vi "OpenGDS_Installer.vi"() -> ()   [LabVIEW 2012]
uses:
  OpenGDS_Installer_State.ctl
  <vilib>/Utility/config.llb/Read Key (String).vi
  <vilib>/zip/NI_Unzip.lvlib
  <vilib>/Utility/config.llb/NI_LVConfig.lvlib
panel:
  out "Tab":enum32{"Full", "Small"}(tab)
  in  "Restart":bool
  out "FullDetailsText":string
  out "FullHeader":string
  out "SmallDetailsText":string
  out "SmallHeaderText":string
  out "SmallSteps":enum32{"License", "Ready?", "Progress"}(tab)
  in  "Accept":bool
  out "Lic":string
  out "Ready?-Text":string
  out "Status:":u8(slide) caption="Removing files" scale=0.0..100.0
  out "ProgressText":string
  in  "Back":bool
  in  "Next":bool
  in  "Cancel":bool
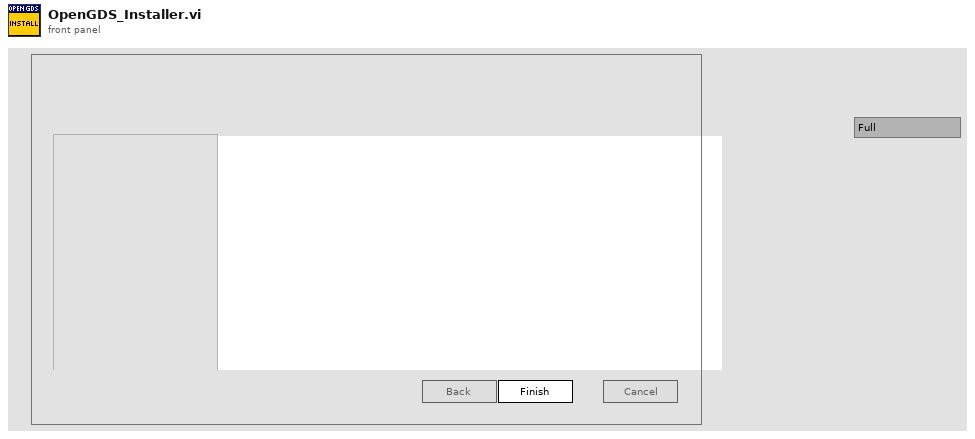
[diagram p1: front panel]
types:
  T1 = typedef "OpenGDS_Installer_State.ctl" = enum16{"Init", "License", "Ready?", "Progress", "Cancelled", "Finished"}
  T2 = cluster{"State":T1, "FilesCopied":i32, "ErrorTest":string, "Files":path[], "ReCompile":bool}
  T3 = typedef "LVRectTypeDef.ctl" = cluster{"Left":i16, "Top":i16, "Right":i16, "Bottom":i16}
  T4 = enum8{"Enabled", "Disabled", "Disabled and Grayed Out"}
  T5 = typedef "NI_LVConfig.lvlib/Config Data RefNum.ctl" = refnum<k1>
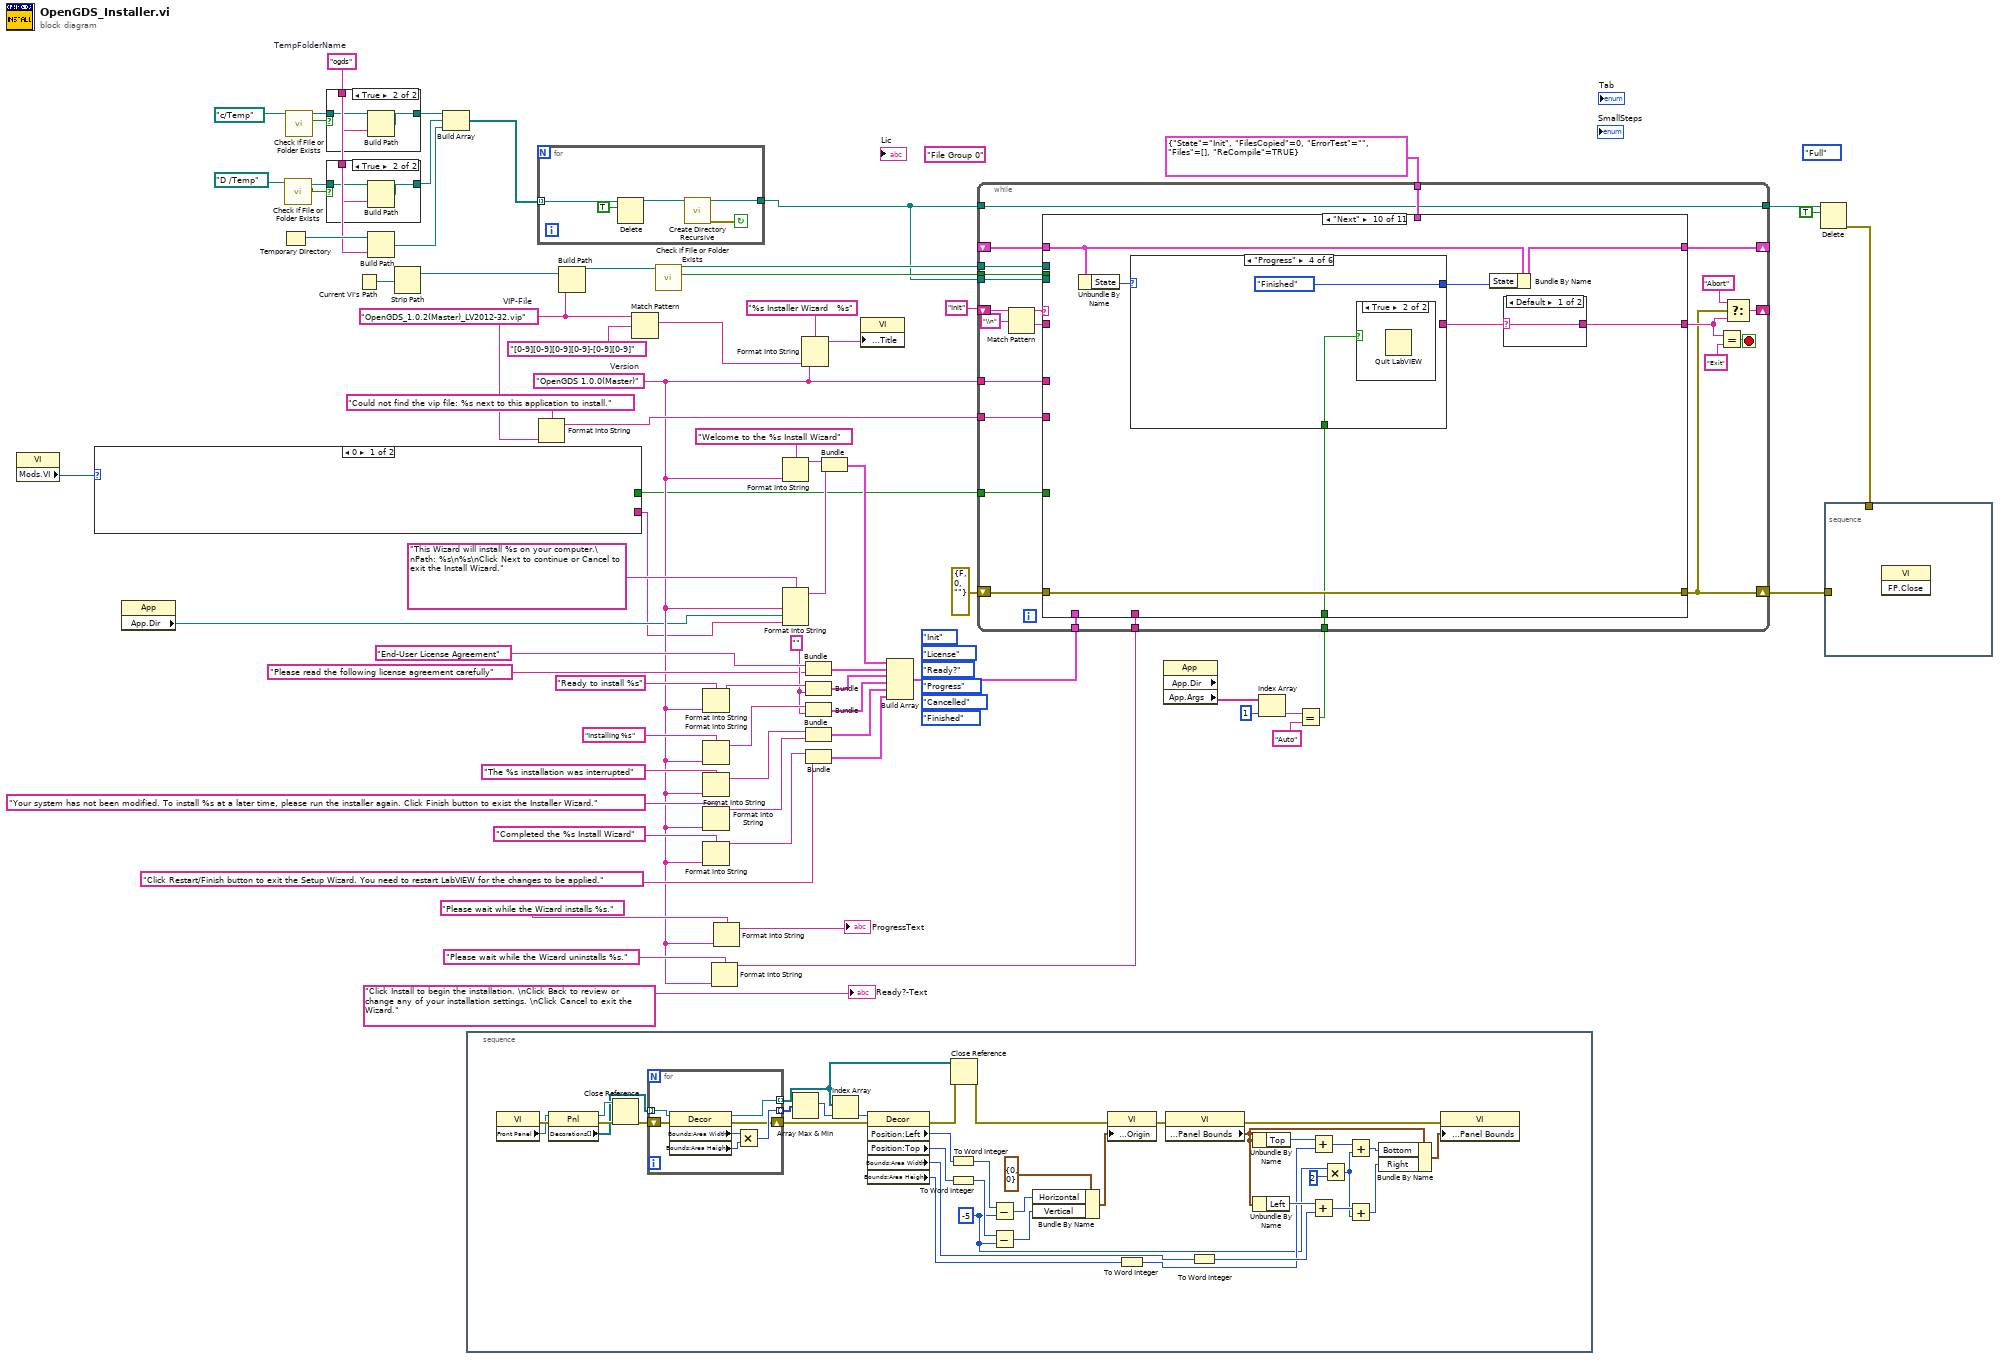
[diagram p0: block diagram]
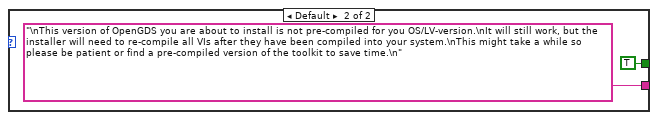
[diagram p4: hidden frame]
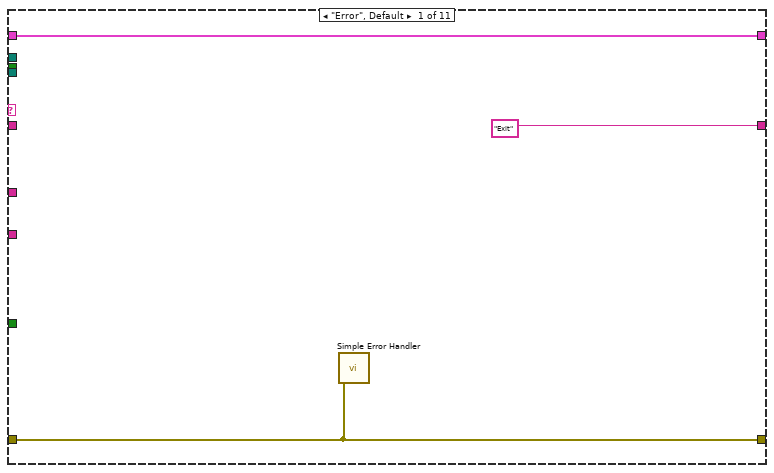
[diagram p5: hidden frame]
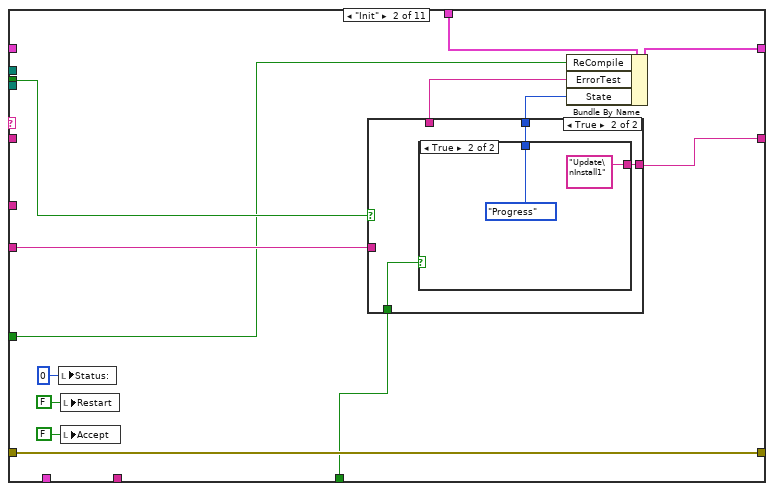
[diagram p6: hidden frame]
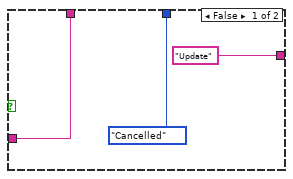
[diagram p7: hidden frame]
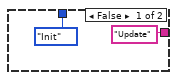
[diagram p8: hidden frame]
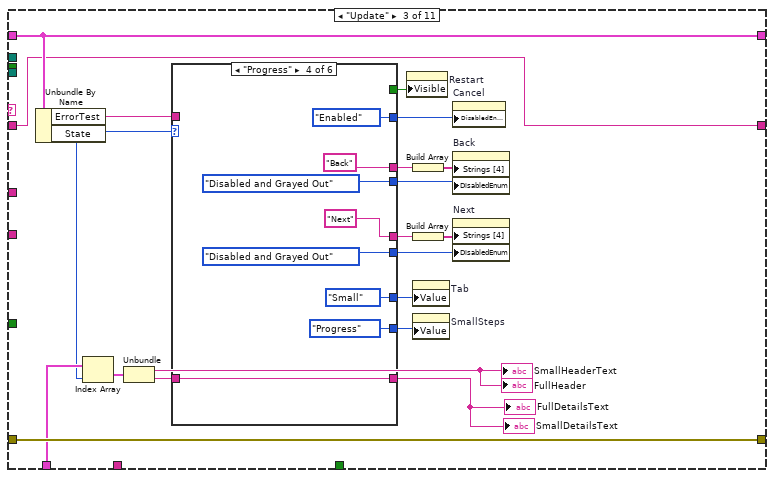
[diagram p9: hidden frame]
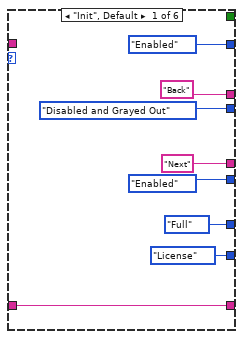
[diagram p10: hidden frame]
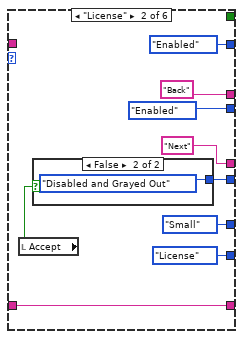
[diagram p11: hidden frame]
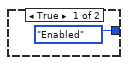
[diagram p12: hidden frame]
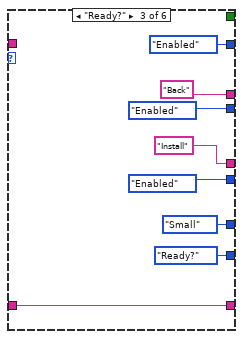
[diagram p13: hidden frame]
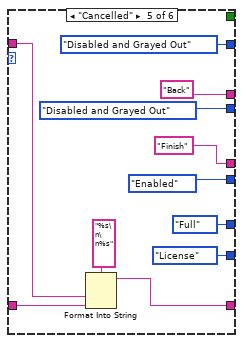
[diagram p14: hidden frame]
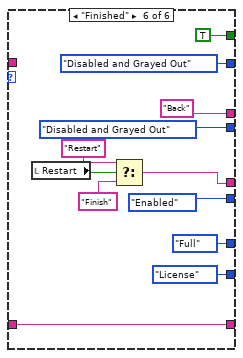
[diagram p15: hidden frame]
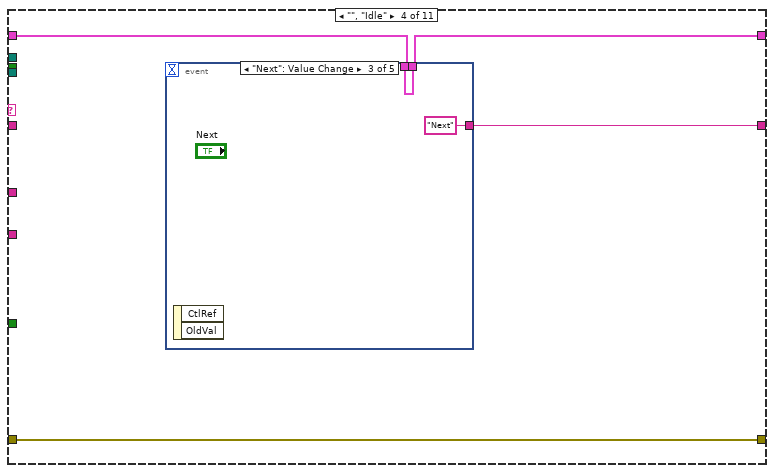
[diagram p16: hidden frame]
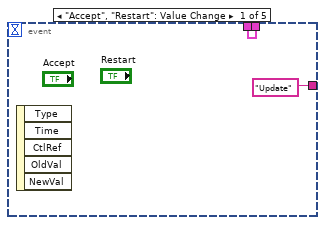
[diagram p17: hidden frame]
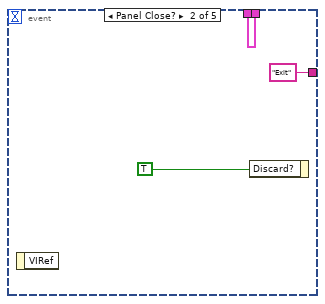
[diagram p18: hidden frame]
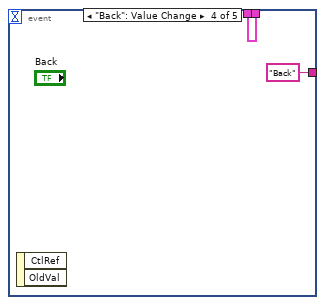
[diagram p19: hidden frame]
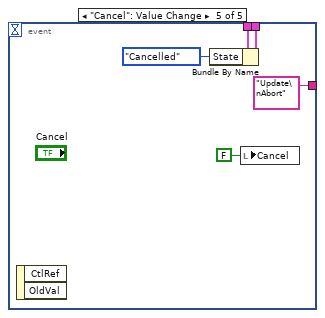
[diagram p20: hidden frame]
diagram:
  w9 = "ogds"  # TempFolderName
  (unwired) "File Group 0" ("section")
  w3 = "OpenGDS_1.0.2(Master)_LV2012-32.vip"  # VIP-File
  w46 = ""
  (unwired) OpenGDS_Installer_State."Finished" ("State")
  (unwired) OpenGDS_Installer_State."Cancelled" ("State")
  (unwired) OpenGDS_Installer_State."Progress" ("State")
  (unwired) OpenGDS_Installer_State."Ready?" ("State")
  (unwired) OpenGDS_Installer_State."License" ("State")
  (unwired) OpenGDS_Installer_State."Init" ("State")
  (unwired) enum32{"Full", "Small"}."Full" ("Tab")
  w32 = "OpenGDS 1.0.0(Master)"  # Version
  n1 = property class="VI"() -> ("Mods.VI"=w24:u64)  [unwired: 2 in, 2 out]
  n2 = case shown="0" w24 {
    tunnel: [_ "\nThis version of OpenGDS you are about to install is not pre-compiled for you OS/LV-version.\nIt will still work, but the installer will need to re-compile all VIs after they have been compiled into your system.\nThis might take a while so please be patient or find a pre-compiled version of the toolkit to save time.\n"] -> w23
    tunnel: [_ TRUE] -> w22
    frame 0 {
    }
    frame Default {
    }
  }
  n3 = property class="App"() -> ("App.Dir"=w29:path)  [unwired: 2 in, 2 out]
  n4 = Temporary Directory() -> (w15:path)
  n5 = call <vilib>:"Check if File or Folder Exists.vi"("path"=path "/D /Temp") -> ("file or folder exists?"=w16:bool, "dup path"=w17:path)  [unwired: 8 in, 1 out]
  n6 = call <vilib>:"Check if File or Folder Exists.vi"("path"=path "c:/Temp") -> ("file or folder exists?"=w19:bool, "dup path"=w18:path)  [unwired: 8 in, 1 out]
  n7 = case shown="True" w19 {
    tunnel: w18 -> [w75 w78]
    tunnel: w9 -> [_ w77]
    tunnel: [w75 w76] -> w14
    frame False {
    }
    frame True {
      n8 = Build Path(base path=w78, name or relative path=w77) -> (appended path=w76:path)
    }
  }
  n9 = case shown="True" w16 {
    tunnel: w17 -> [w79 w82]
    tunnel: w9 -> [_ w81]
    tunnel: [w79 w80] -> w13
    frame False {
    }
    frame True {
      n10 = Build Path(base path=w82, name or relative path=w81) -> (appended path=w80:path)
    }
  }
  n11 = Current VI's Path() -> (path=w40:path)
  n12 = Build Path(base path=w15, name or relative path=w9) -> (appended path=w12:path)
  n13 = Strip Path(path=w40) -> (stripped path=w39:path)  [unwired: 1 out]
  n14 = Build Array(w14, w13, w12) -> (w11:path[])
  n15 = stacked-sequence {
    frame #0 {
      w86 = i16 -5 ("border spacing (2 px)")
      n16 = property on="Property Node" class="VI"() -> (error out=w119:errorcluster, "Front Panel"=w117:refnum<vi>)  [unwired: 2 in, 1 out]
      n17 = property on="Property Node" class="Pnl"(reference=w117, error in=w119) -> (reference out=w120:refnum<vi>, error out=w118:errorcluster, "Decorations[]"=w115:refnum<vi>[])
      n18 = Close Reference(reference=w120, error in (no error)=w118) -> (error out=w116:errorcluster)
      n19 = for {
        tunnel: w115 -> [w127] mode=indexing
        tunnel: [w124] -> w98 mode=indexing
        shift-right: [w122] -> w95
        shift-left: w116 -> [w123]
        tunnel: [w121] -> w85 mode=indexing
        n20 = property class="Decor"(reference=w127, error in=w123) -> (reference out=w121:refnum<vi>, error out=w122:errorcluster, "Bounds:Area Width"=w126:u32, "Bounds:Area Height"=w125:u32)
        n21 = Multiply(x=w126, y=w125) -> (x*y=w124:u32)
      }
      n22 = Array Max & Min(array=w98) -> (max index (indices)=w97:i32)  [unwired: 3 out]
      n23 = Index Array(array=w85, index=w97) -> (element=w96:refnum<vi>)
      n24 = property class="Decor"(reference=w96, error in=w95) -> (error out=w84:errorcluster, "Position:Left"=w101:i32, "Position:Top"=w104:i32, "Bounds:Area Width"=w109:u32, "Bounds:Area Height"=w107:u32)  [unwired: 1 out]
      n25 = To Word Integer(number=w101) -> (16bit integer=w88:i16)
      n26 = To Word Integer(number=w104) -> (16bit integer=w87:i16)
      n27 = Close Reference(reference=w85, error in (no error)=w84) -> (error out=w83:errorcluster)
      n28 = Subtract(x=w88, y=w86) -> (x-y=w102:i16)
      n29 = Subtract(x=w87, y=w86) -> (x-y=w103:i16)
      n30 = Bundle By Name(cluster=cluster{"Horizontal":i16, "Vertical":i16} {"Horizontal"=0, "Vertical"=0} ("Front Panel Window:Origin"), "Horizontal"=w102, "Vertical"=w103) -> (w99:cluster{"Horizontal":i16, "Vertical":i16})
      n31 = property on="Property Node" class="VI"(error in=w83, "Front Panel Window:Origin"=w99) -> (error out=w93:errorcluster)  [unwired: 1 in, 1 out]
      n32 = To Word Integer(number=w107) -> (16bit integer=w89:i16)
      n33 = property on="Property Node" class="VI"(error in=w93) -> (error out=w92:errorcluster, "Front Panel Window:Panel Bounds"=w105:T3)  [unwired: 1 in, 1 out]
      n34 = To Word Integer(number=w109) -> (16bit integer=w90:i16)
      n35 = Unbundle By Name(w105) -> ("Top"=w106:i16)
      n36 = Unbundle By Name(w105) -> ("Left"=w108:i16)
      n37 = Add(x=w106, y=w89) -> (x+y=w113:i16)
      n38 = Add(x=w108, y=w90) -> (x+y=w111:i16)
      n39 = Multiply(x=w86, y=i16 2) -> (x*y=w91:i16)
      n40 = Add(x=w113, y=w91) -> (x+y=w114:i16)
      n41 = Add(x=w111, y=w91) -> (x+y=w112:i16)
      n42 = Bundle By Name(cluster=w105, "Bottom"=w114, "Right"=w112) -> (w110:T3)
      n43 = property on="Property Node" class="VI"(error in=w92, "Front Panel Window:Panel Bounds"=w110) -> ()  [unwired: 1 in, 2 out]
    }
  }
  n44 = for {
    tunnel: [w132] -> w10
    tunnel: w11 -> [w129] mode=indexing
    stop <- w128 continue-if-true
    n45 = Delete(path (use dialog)=w129, entire hierarchy (F)=TRUE) -> (deleted path=w130:path)  [unwired: 3 in, 2 out]
    n46 = call <vilib>:"Create Directory Recursive.vi"("directory"=w130) -> ("error out"=w128:errorcluster, "directory copy"=w132:path)  [unwired: 4 in, 1 out]
  }
  n47 = Format Into String(format string="Could not find the vip file: %s next to this application to install.", w3) -> (resulting string=w34:string)  [unwired: 2 in, 1 out]
  n48 = Build Path(base path=w39, name or relative path=w3) -> (appended path=w38:path)
  n49 = Match Pattern(string=w3, regular expression="[0-9][0-9][0-9][0-9]-[0-9][0-9]") -> (match substring=w1:string)  [unwired: 1 in, 3 out]
  n50 = call <vilib>:"Check if File or Folder Exists.vi"("path"=w38) -> ("file or folder exists?"=w37:bool, "dup path"=w30:path)  [unwired: 8 in, 1 out]
  n51 = Format Into String(format string="Ready to install %s", w32) -> (resulting string=w58:string)  [unwired: 2 in, 1 out]
  n52 = Format Into String(format string="Installing %s", w32) -> (resulting string=w57:string)  [unwired: 2 in, 1 out]
  n53 = Format Into String(format string="The %s installation was interrupted", w32) -> (resulting string=w48:string)  [unwired: 2 in, 1 out]
  n54 = Format Into String(format string="Your system has not been modified. To install %s at a later time, please run the installer again. Click Finish button to exist the Installer Wizard.", w32) -> (resulting string=w47:string)  [unwired: 2 in, 1 out]
  n55 = Format Into String(format string="Completed the %s Install Wizard", w32) -> (resulting string=w51:string)  [unwired: 2 in, 1 out]
  n56 = Format Into String(format string="Please wait while the Wizard uninstalls %s." ("ProgressText"), w32) -> (resulting string=w31:string)  [unwired: 2 in, 1 out]
  n57 = Format Into String(format string="Please wait while the Wizard installs %s." ("ProgressText"), w32) -> (resulting string=→"ProgressText":string)  [unwired: 2 in, 1 out]
  n58 = Format Into String(format string="Welcome to the %s Install Wizard", w32) -> (resulting string=w63:string)  [unwired: 2 in, 1 out]
  n59 = Format Into String(format string="This Wizard will install %s on your computer.\nPath: %s\n%s\nClick Next to continue or Cancel to exit the Install Wizard.", w32, w29, w23) -> (resulting string=w62:string)  [unwired: 2 in, 1 out]
  n60 = Format Into String(format string="%s Installer Wizard   %s", w32, w1) -> (resulting string=w69:string)  [unwired: 2 in, 1 out]
  n61 = Bundle("End-User License Agreement", "Please read the following license agreement carefully") -> (w60:cluster{string, string})  [unwired: 1 in]
  n62 = Bundle(w58, w46) -> (w56:cluster{string, string})  [unwired: 1 in]
  n63 = Bundle(w57, w46) -> (w55:cluster{string, string})  [unwired: 1 in]
  n64 = Bundle(w48, w47) -> (w54:cluster{string, string})  [unwired: 1 in]
  n65 = Bundle(w51, "input 1"="Click Restart/Finish button to exit the Setup Wizard. You need to restart LabVIEW for the changes to be applied.") -> (w53:cluster{string, "input 1":string})  [unwired: 1 in]
  n66 = Bundle(w63, w62) -> (w61:cluster{string, string})  [unwired: 1 in]
  n67 = property on="Property Node" class="VI"("Front Panel.Title"=w69) -> ()  [unwired: 2 in, 2 out]
  n68 = Build Array(w61, w60, w56, w55, w54, w53) -> (w64:cluster{string, "input 1":string}[])
  n69 = property class="App" props=["App.Dir", "App.Args"]() -> ("App.Args"=w5:string[])  [unwired: 2 in, 3 out]
  n70 = Index Array(array=w5, index=1) -> (element=w7:string)
  n71 = Equal?(x=w7, y="Auto") -> (x = y?=w4:bool)
  n72 = while {
    shift-right: [w150] -> w26
    shift-left: errorcluster {"status"=FALSE, "code"=0, "source"=""} ("error IO") -> [w156]
    shift-right: [w155] -> _
    shift-left: "Init" -> [w146]
    shift-right: [w149] -> _
    shift-left: _ -> [w148]
    tunnel: w32 -> [w147]
    tunnel: w64 -> [w142]
    tunnel: w37 -> [w141]
    tunnel: w34 -> [w140]
    tunnel: T2 {"State"=enum."Init", "FilesCopied"=0, "ErrorTest"="", "Files"=[], "ReCompile"=TRUE} -> [w139]
    tunnel: w31 -> [w138]
    tunnel: w30 -> [w137]
    tunnel: w10 -> [w136]
    tunnel: w10 -> [w135]
    tunnel: [w135] -> w28
    tunnel: w22 -> [w134]
    tunnel: w4 -> [w133]
    stop <- w154 stop-if-true
    n73 = Match Pattern(string=w146, regular expression="\\n") -> (before substring=w145:string, after substring=w143:string)  [unwired: 1 in, 2 out]
    n74 = case shown="\"Next\"" w145 {
      tunnel: w156 -> [w157 w172 w201 w261 w292 w326 w353 w402 w485 w499 w519]
      tunnel: [w157 w172 w201 w261 w279 w316 w352 w399 w485 w499 w519] -> w150
      tunnel: ["Exit" w161 w194 w262 "Update" w328 w360 w414 "Next" w500 w520] -> w151
      tunnel: [w158 w171 w202 w263 w288 w330 w362 w400 w487 w503 w523] -> w149
      tunnel: w148 -> [w158 _ w202 w264 w286 w331 w350 w400 w487 w504 w524]
      tunnel: w147 -> [_ _ _ _ _ _ _ _ _ _ _]
      tunnel: w143 -> [_ _ w194 _ _ _ _ _ _ _ _]
      tunnel: w142 -> [_ _ w190 _ _ _ _ _ _ _ _]
      tunnel: w141 -> [_ w168 _ _ _ _ _ _ _ _ _]
      tunnel: w140 -> [_ w167 _ _ _ _ _ _ _ _ _]
      tunnel: w139 -> [_ w165 _ _ _ _ _ _ _ _ _]
      tunnel: w138 -> [_ _ _ _ w284 _ _ _ _ _ _]
      tunnel: w137 -> [_ _ _ _ _ w327 _ _ _ _ _]
      tunnel: w136 -> [_ _ _ _ _ w321 w358 _ _ _ _]
      tunnel: w134 -> [_ w162 _ _ _ _ _ _ _ _ _]
      tunnel: w133 -> [_ w160 _ _ _ _ _ _ _ w497 _]
      frame "Error", Default {
        n75 = call <vilib>:"Simple Error Handler.vi"("error in (no error)"=w157) -> ()  [unwired: 4 in, 5 out]
      }
      frame "Init" {
        n76 = local write "Status:"(u8 0 ("Status:")) -> ()
        n77 = local write "Restart"(FALSE ("Restart")) -> ()
        n78 = local write "Accept"(FALSE ("Accept")) -> ()
        n79 = case shown="True" w168 {
          tunnel: w167 -> [w174 _]
          tunnel: [OpenGDS_Installer_State."Cancelled" ("State") w178] -> w166
          tunnel: [w174 _] -> w164
          tunnel: ["Update" w177] -> w161
          tunnel: w160 -> [_ w176]
          frame False {
          }
          frame True {
            n80 = case shown="True" w176 {
              tunnel: [OpenGDS_Installer_State."Init" ("State") OpenGDS_Installer_State."Progress" ("State")] -> w178
              tunnel: ["Update" "Update\nInstall1"] -> w177
              frame False {
              }
              frame True {
              }
            }
          }
        }
        n81 = Bundle By Name(cluster=w165, "ReCompile"=w162, "ErrorTest"=w164, "State"=w166) -> (w171:T2)
      }
      frame "Update" {
        n82 = Unbundle By Name(w202) -> ("ErrorTest"=w183:string, "State"=w189:T1)
        n83 = Index Array(array=w190, index=w189) -> (element=w187:cluster{string, "input 1":string})
        n84 = Unbundle(w187) -> (→"SmallHeaderText" →"FullHeader":string, "input 1"=w185:string)
        n85 = case shown="\"Progress\"" w189 {
          tunnel: ["Back" "Back" "Back" "Back" "Back" "Back"] -> w198
          tunnel: ["Next" "Next" "Install" "Next" "Finish" w250] -> w197
          tunnel: [T4."Enabled" ("Disabled") w217 T4."Enabled" ("Disabled") T4."Disabled and Grayed Out" ("Disabled") T4."Enabled" ("Disabled") T4."Enabled" ("Disabled")] -> w196
          tunnel: [T4."Disabled and Grayed Out" ("Disabled") T4."Enabled" ("Disabled") T4."Enabled" ("Disabled") T4."Disabled and Grayed Out" ("Disabled") T4."Disabled and Grayed Out" ("Disabled") T4."Disabled and Grayed Out" ("Disabled")] -> w195
          tunnel: [enum32{"Full", "Small"}."Full" ("Tab") enum32{"Full", "Small"}."Small" ("Tab") enum32{"Full", "Small"}."Small" ("Tab") enum32{"Full", "Small"}."Small" ("Tab") enum32{"Full", "Small"}."Full" ("Tab") enum32{"Full", "Small"}."Full" ("Tab")] -> w193
          tunnel: [enum32{"License", "Ready?", "Progress"}."License" ("SmallSteps") enum32{"License", "Ready?", "Progress"}."License" ("SmallSteps") enum32{"License", "Ready?", "Progress"}."Ready?" ("SmallSteps") enum32{"License", "Ready?", "Progress"}."Progress" ("SmallSteps") enum32{"License", "Ready?", "Progress"}."License" ("SmallSteps") enum32{"License", "Ready?", "Progress"}."License" ("SmallSteps")] -> w192
          tunnel: [T4."Enabled" ("Disabled") T4."Enabled" ("Disabled") T4."Enabled" ("Disabled") T4."Enabled" ("Disabled") T4."Disabled and Grayed Out" ("Disabled") T4."Disabled and Grayed Out" ("Disabled")] -> w191
          tunnel: [_ _ _ _ _ TRUE] -> w188
          tunnel: w185 -> [w203 w211 w222 w230 w241 w249]
          tunnel: [w203 w211 w222 w230 w240 w249] -> w184
          tunnel: w183 -> [_ _ _ _ w238 _]
          frame "Init", Default {
          }
          frame "License" {
            n86 = local read "Accept"() -> (w215:bool)
            n87 = case shown="False" w215 {
              tunnel: [T4."Enabled" ("Disabled") T4."Disabled and Grayed Out" ("Disabled")] -> w217
              frame True {
              }
              frame False {
              }
            }
          }
          frame "Ready?" {
          }
          frame "Progress" {
          }
          frame "Cancelled" {
            n88 = Format Into String(format string="%s\n\n%s", w238, w241) -> (resulting string=w240:string)  [unwired: 2 in, 1 out]
          }
          frame "Finished" {
            n89 = local read "Restart"() -> (w253:bool)
            n90 = Select(t="Restart", s=w253, f="Finish") -> (s? t:f=w250:string)
          }
        }
        "FullDetailsText" <- w184
        "SmallDetailsText" <- w184
        n91 = property on="Restart" class="Bool (strict)"("Visible"=w188) -> ()  [unwired: 2 in, 2 out]
        n92 = Build Array(w198) -> (w200:string[])
        n93 = Build Array(w197) -> (w199:string[])
        n94 = property on="Tab" class="TabCtl (strict)"("Value"=w193) -> ()  [unwired: 2 in, 2 out]
        n95 = property on="SmallSteps" class="TabCtl (strict)"("Value"=w192) -> ()  [unwired: 2 in, 2 out]
        n96 = property on="Cancel" class="Bool (strict)"("DisabledEnum"=w191) -> ()  [unwired: 2 in, 2 out]
        n97 = property on="Back" class="Bool"("Strings [4]"=w200, "DisabledEnum"=w195) -> ()  [unwired: 2 in, 2 out]
        n98 = property on="Next" class="Bool"("Strings [4]"=w199, "DisabledEnum"=w196) -> ()  [unwired: 2 in, 2 out]
      }
      frame "", "Idle" {
        n99 = event shown="[2] \"Next\": Value Change" {
          selector: _ -> [_ _ _ _ _]
          dyn-events: _ -> [_ _ _ _ _]
          timeout: _ -> [_ _ _ _ _]
          tunnel: w264 -> [w266 w268 w271 w273 w278]
          tunnel: [w266 w268 w271 w273 w275] -> w263
          tunnel: ["Update" "Exit" "Next" "Back" "Update\nAbort"] -> w262
          event "Accept", "Restart": Value Change {
            n100 = event-data() -> ()  [unwired: 1 in, 5 out]
          }
          event Panel Close? {
            n101 = event-data() -> ()  [unwired: 1 in, 1 out]
            n102 = event-data("Discard?"=TRUE) -> ()  [unwired: 1 in, 1 out]
          }
          event "Next": Value Change {
            n103 = event-data() -> ()  [unwired: 1 in, 2 out]
          }
          event "Back": Value Change {
            n104 = event-data() -> ()  [unwired: 1 in, 2 out]
          }
          event "Cancel": Value Change {
            n105 = event-data() -> ()  [unwired: 1 in, 2 out]
            n106 = Bundle By Name(cluster=w278, "State"=OpenGDS_Installer_State."Cancelled") -> (w275:T2)
            n107 = local write "Cancel"(FALSE ("Cancel")) -> ()
          }
        }
      }
      frame "Abort" {
        # "Remove Files"
        n108 = Unbundle By Name(w286) -> ("Files"=w282:path[], "FilesCopied"=w283:i32)
        n109 = property class="App"() -> ("App.Dir"=w280:path)  [unwired: 2 in, 2 out]
        n110 = local write "Cancel"(FALSE ("Cancel")) -> ()
        n111 = Array Size(array=w282) -> (size(s)=w281:i32)
        n112 = for {
          N: w283 -> [w299]
          tunnel: w282 -> [w298] mode=indexing
          tunnel: w281 -> [w300]
          tunnel: w280 -> [w297]
          i -> [w303]
          n113 = Build Path(base path=w297, name or relative path=w298) -> (appended path=w293:path)
          n114 = Subtract(x=w299, y=w303) -> (x-y=w301:i32)
          n115 = Increment(x=w301) -> (x+1=w304:i32)
          n116 = Path To String(path=w293) -> (string=w295:string)
          n117 = Divide(x=w304, y=w300) -> (x/y=w306:dbl)
          n118 = Match Pattern(string=w295, regular expression="addons") -> (offset past match=w294:i32)  [unwired: 1 in, 3 out]
          n119 = Multiply(x=w306, y=100.0) -> (x*y=w302:dbl)
          n120 = local write "Status:"(w302) -> ()
          n121 = case shown="-1" w294 {
            tunnel: w293 -> [_ w307]
            frame 0, Default {
            }
            frame -1 {
              n122 = Set Permissions(7:i16 511 ("permissions"), 11:w307) -> (0:w309:errorcluster, 3:w308:path)  [unwired: 3 in]
              n123 = Delete(path (use dialog)=w308, error in=w309) -> ()  [unwired: 3 in, 3 out]
            }
          }
        }
        n124 = local write "ProgressText"(w284) -> ()
        n125 = Bundle By Name(cluster=w286, "State"=OpenGDS_Installer_State."Cancelled") -> (w288:T2)
        n126 = property on="Cancel" class="Bool (strict)"("DisabledEnum"=T4."Disabled and Grayed Out" ("Disabled")) -> ()  [unwired: 2 in, 2 out]
        n127 = property on="Status:" class="Slide (strict)"("Caption.Text"="Removing files") -> ()  [unwired: 2 in, 2 out]
        n128 = call <vilib>:"Clear Errors.vi"("error in (no error)"=w292) -> ("error out"=w279:errorcluster)  [unwired: 6 in]
      }
      frame "Install1" {
        n129 = call <vilib>:"Unzip.vi"("error in (no error)"=w326, "Target directory (same as Zip file if empty)"=w321, "Zip file"=w327) -> ("error out"=w318:errorcluster)  [unwired: 6 in, 2 out]
        n130 = Build Path(base path=w321, name or relative path="spec") -> (appended path=w319:path)
        n131 = call <vilib>:"Open Config Data.vi"("error in (no error)"=w318, "create file if necessary (T)"=FALSE, "configuration file path"=w319) -> ("error out"=w323:errorcluster, "refnum"=w325:T5)  [unwired: 6 in, 1 out]
        n132 = while {
          shift-right: [w336] -> w324
          shift-left: w323 -> [w343]
          tunnel: w325 -> [w342]
          tunnel: [w332] -> w317 mode=indexing if=w337
          tunnel: [w334] -> w315
          i -> [w341]
          stop <- w335 continue-if-true
          n133 = Format Into String(format string="File %d", w341) -> (resulting string=w339:string)  [unwired: 2 in, 1 out]
          n134 = local read "Cancel"() -> (w334:bool)
          n135 = call-poly <vilib>:"Read Key.vi"("section"="File Group 0", "error in (no error)"=w343, "key"=w339, "refnum"=w342) -> ("error out"=w336:errorcluster, "value"=w333:string, "found?"=w337:bool)  [unwired: 4 in, 1 out]
          n136 = String To Path(string=w333) -> (path=w332:path)
          n137 = Compound Arithmetic op=AND(w337, invert w336, invert w334) -> (w335:bool)
        }
        n138 = property on="Status:" class="Slide (strict)"("Caption.Text"="Unzipping Files") -> ()  [unwired: 2 in, 2 out]
        n139 = local write "Status:"(u8 0 ("Status:")) -> ()
        n140 = call <vilib>:"Close Config Data.vi"("error in (no error)"=w324, "refnum"=w325) -> ("error out"=w316:errorcluster)  [unwired: 8 in, 1 out]
        n141 = Bundle By Name(cluster=w331, "FilesCopied"=0, "Files"=w317) -> (w330:T2)
        n142 = Select(t="Abort", s=w315, f="Install2") -> (s? t:f=w328:string)
      }
      frame "Install2" {
        n143 = Build Path(base path=w358, name or relative path="File Group 0" ("section")) -> (appended path=w356:path)
        n144 = property class="App"() -> ("App.Dir"=w354:path)  [unwired: 2 in, 2 out]
        n145 = property on="Status:" class="Slide (strict)"("Caption.Text"="Copying files") -> ()  [unwired: 2 in, 2 out]
        n146 = Unbundle By Name(w350) -> ("Files"=w355:path[])
        n147 = Unbundle By Name(w350) -> ("ReCompile"=w346:bool)
        n148 = for {
          N -> [w379]
          shift-right: [w369] -> w352
          shift-left: w353 -> [w386]
          tunnel: w356 -> [w374]
          tunnel: w355 -> [w371] mode=indexing
          tunnel: w354 -> [w372]
          tunnel: [w368] -> w344
          tunnel: [w365] -> w351
          tunnel: w346 -> [w364]
          tunnel: [w363] -> w345 mode=indexing
          i -> [w367]
          stop <- w366 stop-if-true
          n149 = Build Path(base path=w372, name or relative path=w371) -> (appended path=w370:path)
          n150 = Build Path(base path=w374, name or relative path=w371) -> (appended path=w373:path)
          n151 = Strip Path(path=w370) -> (stripped path=w387:path)  [unwired: 1 out]
          n152 = call <vilib>:"Create Directory Recursive.vi"("error in (no error)"=w386, "directory"=w387) -> ("error out"=w385:errorcluster)  [unwired: 3 in, 2 out]
          n153 = call <vilib>:"Check if File or Folder Exists.vi"("error in (no error)"=w385, "path"=w370) -> ("error out"=w384:errorcluster, "file or folder exists?"=w381:bool, "dup path"=w383:path)  [unwired: 7 in]
          n154 = Increment(x=w367) -> (x+1=w365:i32)
          n155 = Divide(x=w365, y=w379) -> (x/y=w378:dbl)
          n156 = case shown="True" w381 {
            tunnel: w384 -> [w393 w397]
            tunnel: w383 -> [_ w396]
            tunnel: [w393 w394] -> w382
            frame False {
            }
            frame True {
              n157 = Set Permissions(7:i16 511 ("permissions"), 8:w397, 11:w396) -> (0:w394:errorcluster)  [unwired: 2 in, 1 out]
            }
          }
          n158 = Multiply(x=w378, y=100.0) -> (x*y=→"Status:":dbl)
          n159 = local read "Cancel"() -> (w368:bool)
          n160 = Copy(8:w382, 9:TRUE ("overwrite (F)"), 10:w370, 11:w373) -> (0:w376:errorcluster, 3:w363:path)  [unwired: 1 in, 1 out]
          n161 = case shown="True" w364 {
            tunnel: w363 -> [w390 _]
            tunnel: w376 -> [w389 w392]
            tunnel: [w388 w392] -> w369
            frame False {
              n162 = Set Permissions(7:i16 365 ("permissions"), 8:w389, 11:w390) -> (0:w388:errorcluster)  [unwired: 2 in, 1 out]
            }
            frame True {
            }
          }
          n163 = Or(x=w369, y=w368) -> (x .or. y?=w366:bool)
        }
        n164 = Bundle By Name(cluster=w350, "FilesCopied"=w351, "Files"=w345) -> (w362:T2)
        n165 = Select(t="ReCompile1", s=w346, f="Next") -> (s? t:f=w348:string)
        n166 = Select(t="Abort", s=w344, f=w348) -> (s? t:f=w360:string)
      }
      frame "ReCompile1" {
        n167 = Unbundle By Name(w400) -> ("Files"=w401:path[])
        n168 = property on="Status:" class="Slide (strict)"("Caption.Text"="Re-compiling") -> ()  [unwired: 2 in, 2 out]
        n169 = for {
          N -> [w438]
          tunnel: [w450] -> w407 mode=concatenating if=w449
          shift-right: [w436] -> w403
          shift-left: w402 -> [w443]
          tunnel: [w448] -> w409 mode=indexing if=w447
          tunnel: [w446] -> w410 mode=indexing if=w445
          tunnel: w401 -> [w434] mode=indexing
          tunnel: [w433] -> w398
          i -> [w439]
          stop <- w435 stop-if-true
          n170 = call <vilib>:"Get File Extension.vi"("error in (no error)"=w443, "file"=w434) -> ("error out"=w444:errorcluster, "lowercase file extension"=w452:string, "dup file"=w451:path)  [unwired: 6 in, 1 out]
          n171 = case shown="\"ctl\", \"vi\", \"vit\"" w452 {
            tunnel: w444 -> [w453 w460 w465 w470 w472]
            tunnel: w451 -> [_ w459 w464 w469 w471]
            tunnel: [_ w455 _ _ w477] -> w450
            tunnel: [_ TRUE _ _ TRUE] -> w449
            tunnel: [w453 w456 w463 w466 w475] -> w436
            tunnel: [_ _ _ w468 _] -> w448
            tunnel: [_ _ _ TRUE _] -> w447
            tunnel: [_ _ w462 _ _] -> w446
            tunnel: [_ _ TRUE _ _] -> w445
            frame Default {
            }
            frame "ctl", "vi", "vit" {
              n172 = Open VI Reference(vi path=w459, options=2, error in (no error)=w460) -> (vi reference=w458:refnum<vi>, error out=w456:errorcluster)  [unwired: 3 in]
              n173 = Build Array(w458) -> (w455:refnum<vi>[])
            }
            frame "lvclass" {
              n174 = invoke class="App" method="LVClass.Open"(error in=w465, "Path"=w464) -> (error out=w463:errorcluster, "LVClass.Open"=w462:refnum<vi>)  [unwired: 2 in, 2 out]
            }
            frame "lvlib" {
              n175 = invoke class="App" method="Library.Open"(error in=w470, "path"=w469) -> (error out=w466:errorcluster, "Open Library"=w468:refnum<vi>)  [unwired: 2 in, 2 out]
            }
            frame "llb" {
              n176 = List Folder(path=w471, error in=w472) -> (filenames=w473:string[], error out=w474:errorcluster)  [unwired: 1 in, 3 out]
              n177 = for {
                tunnel: w473 -> [w478] mode=indexing
                tunnel: w471 -> [w483]
                shift-right: [w480] -> w475
                shift-left: w474 -> [w481]
                tunnel: [w479] -> w477 mode=indexing
                n178 = Build Path(base path=w483, name or relative path=w478) -> (appended path=w482:path)
                n179 = Open VI Reference(vi path=w482, error in (no error)=w481) -> (vi reference=w479:refnum<vi>, error out=w480:errorcluster)  [unwired: 4 in]
              }
            }
          }
          n180 = Increment(x=w439) -> (x+1=w441:i32)
          n181 = Divide(x=w441, y=w438) -> (x/y=w440:dbl)
          n182 = Multiply(x=w440, y=20.0) -> (x*y=w442:dbl)
          n183 = local write "Status:"(w442) -> ()
          n184 = local read "Cancel"() -> (w433:bool)
          n185 = Or(x=w436, y=w433) -> (x .or. y?=w435:bool)
        }
        n186 = for {
          N -> [w426]
          tunnel: w407 -> [w432] mode=indexing
          shift-right: [w430] -> w404
          shift-left: w403 -> [w431]
          i -> [w425]
          n187 = invoke class="VI" method="Save.Instrument"(reference=w432, error in=w431) -> (error out=w430:errorcluster)  [unwired: 4 in, 5 out]
          n188 = Increment(x=w425) -> (x+1=w427:i32)
          n189 = Divide(x=w427, y=w426) -> (x/y=w428:dbl)
          n190 = Multiply(x=w428, y=80.0) -> (x*y=w424:dbl)
          n191 = Add(x=w424, y=20.0) -> (x+y=w422:dbl)
          n192 = local write "Status:"(w422) -> ()
        }
        n193 = for {
          tunnel: w409 -> [w421] mode=indexing
          shift-right: [w419] -> w405
          shift-left: w404 -> [w420]
          n194 = invoke class="Library" method="Save"(reference=w421, error in=w420) -> (error out=w419:errorcluster)  [unwired: 2 in, 3 out]
        }
        n195 = for {
          tunnel: w410 -> [w418] mode=indexing
          shift-right: [w416] -> w406
          shift-left: w405 -> [w417]
          n196 = invoke class="LVClassLibrary" method="Save"(reference=w418, error in=w417) -> (error out=w416:errorcluster)  [unwired: 2 in, 3 out]
        }
        n197 = Close Reference(reference=w407, error in (no error)=w406) -> (error out=w408:errorcluster)
        n198 = Close Reference(reference=w409, error in (no error)=w408) -> (error out=w411:errorcluster)
        n199 = Close Reference(reference=w410, error in (no error)=w411) -> (error out=w399:errorcluster)
        n200 = Select(t="Abort", s=w398, f="ReCompile2") -> (s? t:f=w414:string)
      }
      frame "ReCompile2" {
        n201 = Unbundle By Name(w487) -> ("Files"=w488:path[])
        n202 = for {
          N -> [w489]
          tunnel: w488 -> [w495] mode=indexing
          i -> [w490]
          n203 = Increment(x=w490) -> (x+1=w493:i32)
          n204 = Set Permissions(7:i16 365 ("permissions"), 11:w495) -> ()  [unwired: 3 in, 2 out]
          n205 = Divide(x=w493, y=w489) -> (x/y=w492:dbl)
          n206 = Multiply(x=w492, y=100.0) -> (x*y=w494:dbl)
          n207 = local write "Status:"(w494) -> ()
        }
        n208 = property on="Status:" class="Slide (strict)"("Caption.Text"="Setting file permissions") -> ()  [unwired: 2 in, 2 out]
      }
      frame "Next" {
        n209 = Unbundle By Name(w504) -> ("State"=w502:T1)
        n210 = case shown="\"Progress\"" w502 {
          tunnel: [OpenGDS_Installer_State."License" ("State") OpenGDS_Installer_State."Ready?" ("State") OpenGDS_Installer_State."Progress" ("State") OpenGDS_Installer_State."Finished" ("State") OpenGDS_Installer_State."Cancelled" ("State") OpenGDS_Installer_State."Finished" ("State")] -> w501
          tunnel: [_ _ "Update\nInstall1" _ "Exit" "Exit"] -> w498
          tunnel: w497 -> [_ _ _ w511 _ _]
          frame "Init", Default {
          }
          frame "License" {
          }
          frame "Ready?" {
          }
          frame "Progress" {
            n211 = case shown="True" w511 {
              frame False {
              }
              frame True {
                n212 = Quit LabVIEW() -> ()  [unwired: 1 in]
              }
            }
          }
          frame "Cancelled" {
          }
          frame "Finished" {
            n213 = local read "Restart"() -> (w515:bool)
            n214 = case shown="False" w515 {
              frame False {
              }
              frame True {
                n215 = invoke class="App" method="Restart"() -> ()  [unwired: 3 in, 3 out]
              }
            }
          }
        }
        n216 = Bundle By Name(cluster=w504, "State"=w501) -> (w503:T2)
        n217 = case shown="Default" w498 {
          selector: w498 -> [w505 _]
          tunnel: [w505 "Update"] -> w500
          frame Default {
          }
          frame "" {
          }
        }
      }
      frame "Back" {
        n218 = Unbundle By Name(w524) -> ("State"=w522:T1)
        n219 = case shown="\"Init\", Default" w522 {
          tunnel: [OpenGDS_Installer_State."Init" ("State") OpenGDS_Installer_State."Init" ("State") OpenGDS_Installer_State."License" ("State") OpenGDS_Installer_State."Progress" ("State") OpenGDS_Installer_State."Cancelled" ("State") OpenGDS_Installer_State."Finished" ("State")] -> w521
          tunnel: [_ _ _ _ "Exit" "Exit"] -> w518
          frame "Init", Default {
          }
          frame "License" {
          }
          frame "Ready?" {
          }
          frame "Progress" {
          }
          frame "Cancelled" {
          }
          frame "Finished" {
          }
        }
        n220 = Bundle By Name(cluster=w524, "State"=w521) -> (w523:T2)
        n221 = case shown="Default" w518 {
          selector: w518 -> [w525 _]
          tunnel: [w525 "Update"] -> w520
          frame Default {
          }
          frame "" {
          }
        }
      }
    }
    n222 = Equal?(x=w151, y="Exit") -> (x = y?=w154:bool)
    n223 = Select(t="Abort", s=w150, f=w151) -> (s? t:f=w155:string)
  }
  n224 = Delete(path (use dialog)=w28, entire hierarchy (F)=TRUE) -> (error out=w25:errorcluster)  [unwired: 3 in, 2 out]
  n225 = stacked-sequence {
    tunnel: w26 -> [_]
    tunnel: w25 -> [_]
    frame #0 {
      n226 = invoke class="VI" method="FP.Close"() -> ()  [unwired: 3 in, 3 out]
    }
  }
  "Ready?-Text" <- "Click Install to begin the installation. \nClick Back to review or change any of your installation settings. \nClick Cancel to exit the Wizard." ("ProgressText")
